vi "F Dwf Analog Impedance Mode Get.vi"(8 "error in (no error)":errorcluster, 10 "mode":i32, 11 "hdwf":i32) -> (0 "error out":errorcluster, 2 "mode out":i32, 3 "function return":i32)   [LabVIEW 2019, in "Olasdwf.lvlib"]
doc: "DWFAPI int FDwfAnalogImpedanceModeSet(HDWF hdwf, int mode); DWFAPI int FDwfAnalogImpedanceModeGet(HDWF hdwf, int *mode);"
uses:
  Olasdwf.lvlib
  Windows/System32/dwf.dll
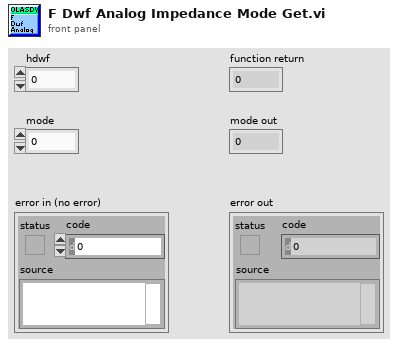
[diagram p1: front panel]
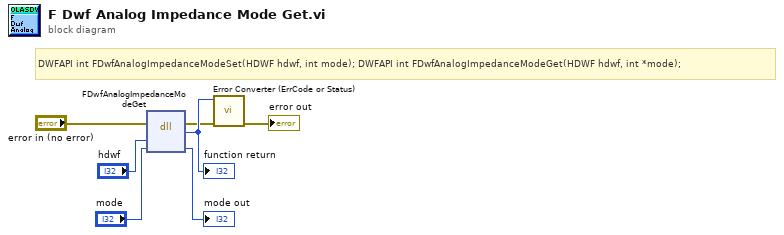
[diagram p0: block diagram]
diagram:
  # "DWFAPI int FDwfAnalogImpedanceModeSet(HDWF hdwf, int mode); DWFAPI int FDwfAnalogImpedanceModeGet(HDWF hdwf, int *mode);"
  n1 = dll-call lib="C:/Windows/System32/dwf.*" fn="FDwfAnalogImpedanceModeGet"(error in="error in (no error)", "hdwf"="hdwf", "mode"="mode") -> (error out=w2:errorcluster, w7:i32, "mode"=→"mode out":i32)  [unwired: 3 in, 1 out]
  "function return" <- w7
  n2 = call "Error Converter (ErrCode or Status).vi"("error in (no error)"=w2, "error code"=w7) -> ("error out"=→"error out":errorcluster)  [unwired: 9 in]
